vi "BRig_Host_dataRunState_typeSelResult_v3.vi"(0 "input_iSelection":u16, 1 "input_LorR":u16, 3 "input_dataPlot":u16[][](array[numeric]), 4 "input_dataTS":u16[][](array[numeric]), 5 "input_idx":i32[](array[numeric]), 6 "input_tSelection":u16, 7 "input_threshold_1":u16, 8 "input_sSelection":u16, 9 "input_threshold_2":u16, 10 "input_nTrial":u16, 14 "input_trig_l2":u16, 15 "input_trig_l1":u16) -> (13 "output_updatePlot":bool, 17 "output_dataPlot":u16[][](array[numeric]), 18 "output_dataTS":u16[][](array[numeric]), 19 "output_idx":i32[](array[numeric]))   [LabVIEW 2014]
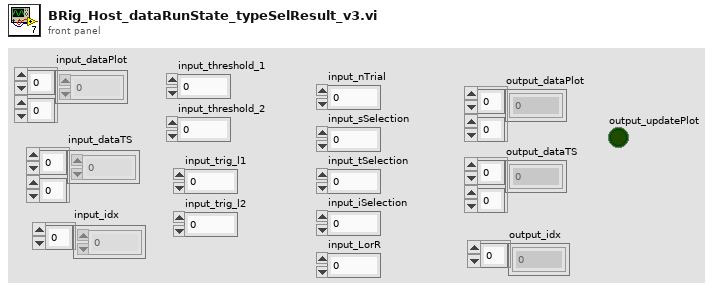
[diagram p1: front panel]
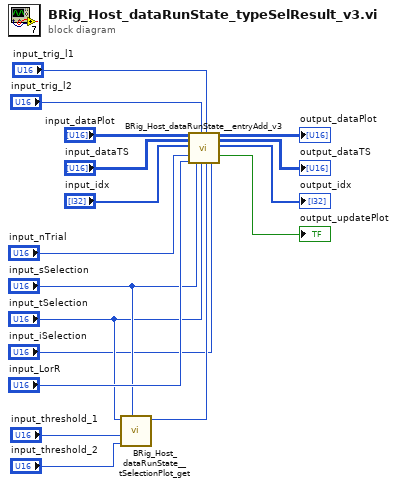
[diagram p0: block diagram]
diagram:
  n1 = call "BRig_Host_dataRunState__tSelectionPlot_get.vi"("input_sSelection"="input_sSelection", "input_threshold_2"="input_threshold_2", "input_threshold_1"="input_threshold_1", "input_tSelection"="input_tSelection") -> ("output_tSelection_plot"=w4:u16)  [unwired: 7 in]
  n2 = call "BRig_Host_dataRunState__entryAdd_v3.vi"("input_dataPlot"="input_dataPlot", "input_dataTS"="input_dataTS", "input_idx"="input_idx", "input_nTrial"="input_nTrial", "input_LorR"="input_LorR", "input_sSelection"="input_sSelection", "input_trig_l2"="input_trig_l2", "input_tSelection"="input_tSelection", "input_trig_l1"="input_trig_l1", "input_tSelectionPlot"=w4, "input_iSelection"="input_iSelection") -> ("output_dataPlot"=→"output_dataPlot":u16[][], "output_dataTS"=→"output_dataTS":u16[][], "output_idx"=→"output_idx":i32[], "output_updatePlot"=→"output_updatePlot":bool)  [unwired: 5 in]
